vi "set_Par_DC.vi"(0 "Autorange":bool, 1 "Voltmeter PLC":dbl=1.0 min=0.01 max=60.0 step=0.01 format="%.2f", 2 "Voltage Compliance":dbl=10.0 min=0.1 max=105.0 step=0.1 format="%.2f", 3 "Address":string="24") -> ()   [LabVIEW 2012]
panel:
  # "ON"
  # "OFF"
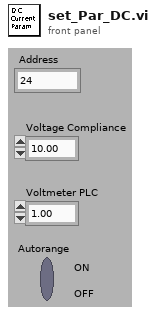
[diagram p1: front panel]
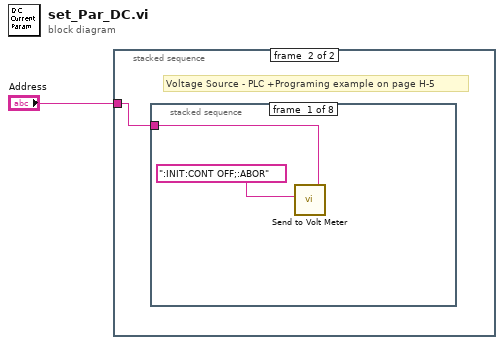
[diagram p0: block diagram]
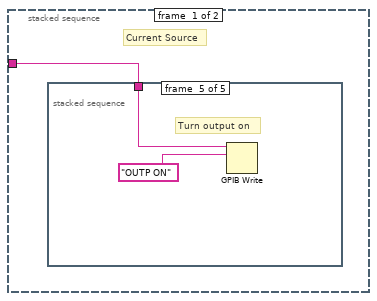
[diagram p2: hidden frame]
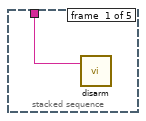
[diagram p3: hidden frame]
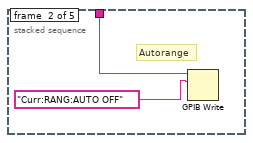
[diagram p4: hidden frame]
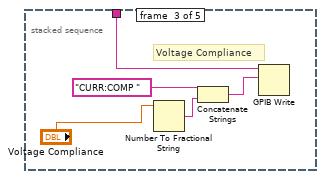
[diagram p5: hidden frame]
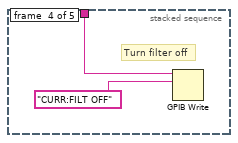
[diagram p6: hidden frame]
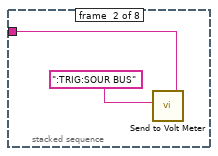
[diagram p7: hidden frame]
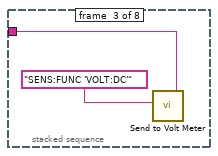
[diagram p8: hidden frame]
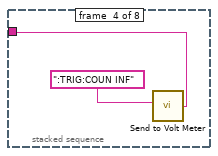
[diagram p9: hidden frame]
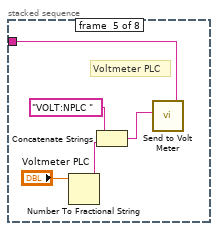
[diagram p10: hidden frame]
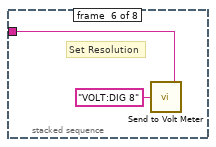
[diagram p11: hidden frame]
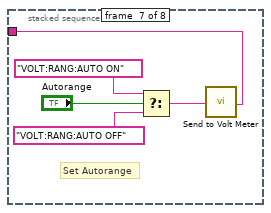
[diagram p12: hidden frame]
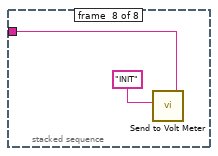
[diagram p13: hidden frame]
diagram:
  n1 = stacked-sequence {
    tunnel: "Address" -> [w2 w15]
    frame #0 {
      # "Current Source"
      n2 = stacked-sequence {
        tunnel: w2 -> [w3 w5 w10 w11 w13]
        frame #0 {
          n3 = call "disarm.vi"("address string"=w3) -> ()  [unwired: 1 in, 1 out]
        }
        frame #1 {
          # "Autorange"
          n4 = GPIB Write(0:w5, 1:"Curr:RANG:AUTO OFF" ("data")) -> ()  [unwired: 3 in, 2 out]
        }
        frame #2 {
          # "Voltage Compliance"
          n5 = Number To Fractional String(number="Voltage Compliance") -> (F-format string=w7:string)  [unwired: 3 in]
          n6 = Concatenate Strings("CURR:COMP " ("data"), w7) -> (w8:string)
          n7 = GPIB Write(0:w10, 1:w8) -> ()  [unwired: 3 in, 2 out]
        }
        frame #3 {
          # "Turn filter off"
          n8 = GPIB Write(0:w11, 1:"CURR:FILT OFF" ("data")) -> ()  [unwired: 3 in, 2 out]
        }
        frame #4 {
          # "Turn output on"
          n9 = GPIB Write(0:w13, 1:"OUTP ON" ("data")) -> ()  [unwired: 3 in, 2 out]
        }
      }
    }
    frame #1 {
      # "Voltage Source - PLC +Programing example on page H-5"
      n10 = stacked-sequence {
        tunnel: w15 -> [w16 w18 w20 w22 w24 w30 w35 w36]
        frame #0 {
          n11 = call "Send to Volt Meter.vi"("Address"=w16, "Data"=":INIT:CONT OFF;:ABOR") -> ()
        }
        frame #1 {
          n12 = call "Send to Volt Meter.vi"("Address"=w18, "Data"=":TRIG:SOUR BUS") -> ()
        }
        frame #2 {
          n13 = call "Send to Volt Meter.vi"("Address"=w20, "Data"="SENS:FUNC 'VOLT:DC'") -> ()
        }
        frame #3 {
          n14 = call "Send to Volt Meter.vi"("Address"=w22, "Data"=":TRIG:COUN INF") -> ()
        }
        frame #4 {
          # "Voltmeter PLC"
          n15 = Number To Fractional String(number="Voltmeter PLC") -> (F-format string=w26:string)  [unwired: 3 in]
          n16 = Concatenate Strings("VOLT:NPLC " ("Data"), w26) -> (w27:string)
          n17 = call "Send to Volt Meter.vi"("Address"=w24, "Data"=w27) -> ()
        }
        frame #5 {
          # "Set Resolution"
          n18 = call "Send to Volt Meter.vi"("Address"=w30, "Data"="VOLT:DIG 8") -> ()
        }
        frame #6 {
          # "Set Autorange"
          n19 = Select(t="VOLT:RANG:AUTO ON", s="Autorange", f="VOLT:RANG:AUTO OFF") -> (s? t:f=w34:string)
          n20 = call "Send to Volt Meter.vi"("Address"=w35, "Data"=w34) -> ()
        }
        frame #7 {
          n21 = call "Send to Volt Meter.vi"("Address"=w36, "Data"="INIT") -> ()
        }
      }
    }
  }
